vi "Adjust Coordinate.vi"(9 "Y":dbl, 10 "X":dbl, 11 "Resolution":i32=444) -> (2 "Offset Only":cluster{dbl, dbl}, 3 "Adjusted Coordinate":cluster{dbl, dbl})   [LabVIEW 2019]
doc: "This VI adjusts a coordinate by incorporating the sample size and offset."
uses:
  Global Variables.vi
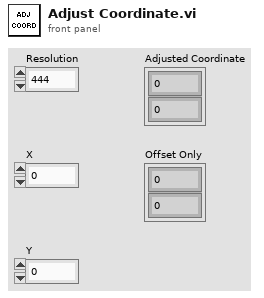
[diagram p1: front panel]
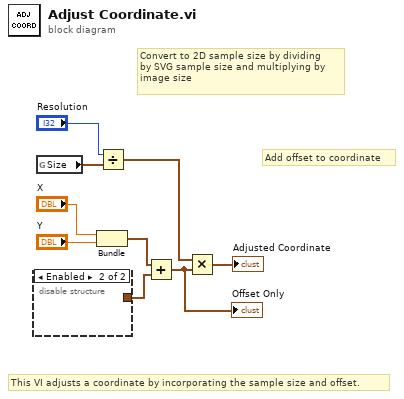
[diagram p0: block diagram]
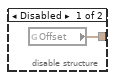
[diagram p2: hidden frame]
diagram:
  # "Add offset to coordinate"
  # "Convert to 2D sample size by dividing\nby SVG sample size and multiplying by\nimage size"
  # "This VI adjusts a coordinate by incorporating the sample size and offset."
  n1 = disable-structure shown="Enabled" {
    disable-tunnel: [w10 _] -> w1
    frame Disabled {
      n2 = global read "Global Variables.vi" "Offset"() -> (w10:cluster{"Width":dbl, "Height":dbl})
    }
    frame Enabled {
    }
  }
  n3 = global read "Global Variables.vi" "Size"() -> (w4:cluster{"Width":dbl, "Height":dbl})
  n4 = Bundle("X"="X", "Y"="Y") -> (w8:cluster{"X":dbl, "Y":dbl})  [unwired: 1 in]
  n5 = Divide(x="Resolution", y=w4) -> (x/y=w2:cluster{"Width":dbl, "Height":dbl})
  n6 = Add(x=w8, y=w1) -> (x+y=w9:cluster{dbl, dbl})
  "Offset Only" <- w9
  n7 = Multiply(x=w2, y=w9) -> (x*y=→"Adjusted Coordinate":cluster{dbl, dbl})
